vi "PIDF.vi"(4 "reinitialize? (F)":bool, 5 "invert? (F)":bool, 6 "PIDF gains":cluster{"Kp":dbl, "Ki":dbl, "Kd":dbl, "Kf":dbl} {"Kf" format="%.3f"; "Kd" format="%.3f"; "Ki" format="%.3f"; "Kp" format="%.3f"}, 7 "output range":cluster{"output high":dbl, "output low":dbl}={"output high"=1.0, "output low"=-1.0} {"output low" format="%.2f"; "output high" format="%.2f"}, 8 "i Zone":dbl=inf format="%.2f", 10 "process variable":dbl format="%.2f", 11 "setpoint":dbl format="%.2f") -> (1 "In i Zone?":bool, 2 "In Range?":bool, 3 "output":dbl format="%.2f")   [LabVIEW 2016]
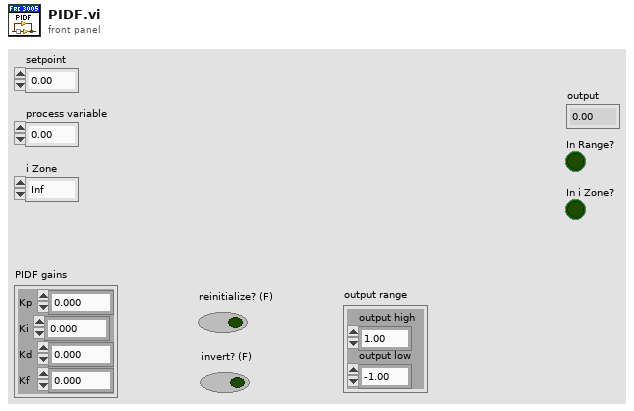
[diagram p1: front panel]
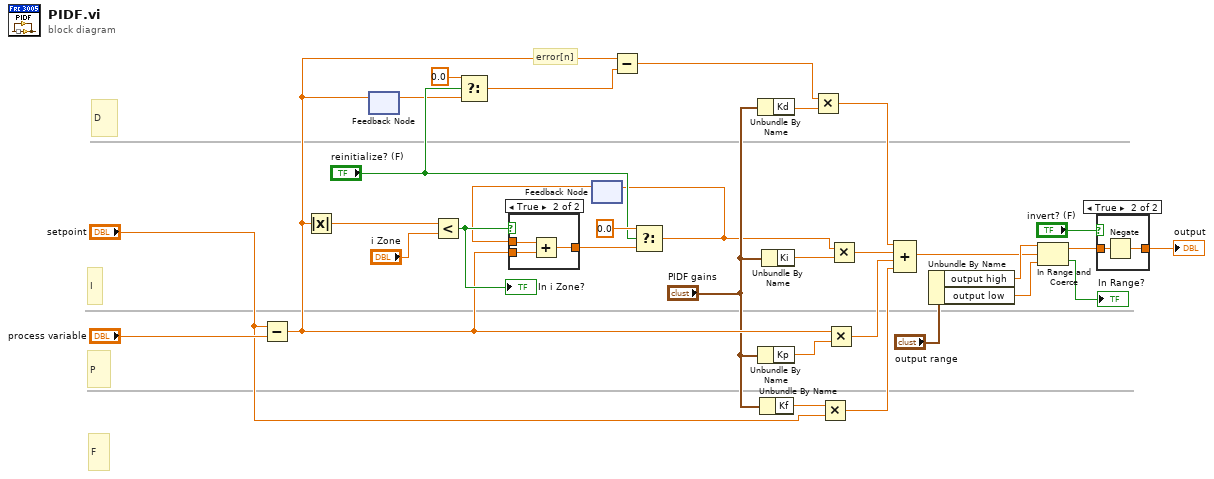
[diagram p0: block diagram]
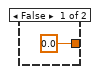
[diagram p3: hidden frame]
diagram:
  # "F"
  # "D"
  # "I"
  # "P"
  # "error[n]"
  n1 = Subtract(x="setpoint", y="process variable") -> (x-y=w23:dbl)
  n2 = Absolute Value(x=w23) -> (abs(x)=w30:dbl)
  n3 = feedback #1() -> (w21:dbl)  [unwired: 1 in]
  n4 = feedback-in #1(w23) -> ()
  n5 = Less?(x=w30, y="i Zone") -> (x < y?=w28:bool)
  "In i Zone?" <- w28
  n6 = Select(t=0.0 ("f"), s="reinitialize? (F)", f=w21) -> (s? t:f=w20:dbl)
  n7 = feedback #2() -> (w27:dbl)  [unwired: 1 in]
  n8 = case shown="True" w28 {
    tunnel: w23 -> [_ w36]
    tunnel: [0.0 ("f") w35] -> w26
    tunnel: w27 -> [_ w34]
    frame False {
    }
    frame True {
      n9 = Add(x=w34, y=w36) -> (x+y=w35:dbl)
    }
  }
  n10 = Subtract(x=w23, y=w20) -> (x-y=w10:dbl)
  n11 = Select(t=0.0 ("f"), s="reinitialize? (F)", f=w26) -> (s? t:f=w7:dbl)
  n12 = feedback-in #2(w7) -> ()
  n13 = Unbundle By Name("PIDF gains") -> ("Kd"=w11:dbl)
  n14 = Unbundle By Name("PIDF gains") -> ("Kp"=w31:dbl)
  n15 = Unbundle By Name("PIDF gains") -> ("Kf"=w13:dbl)
  n16 = Unbundle By Name("PIDF gains") -> ("Ki"=w8:dbl)
  n17 = Multiply(x=w10, y=w11) -> (x*y=w9:dbl)
  n18 = Multiply(x=w13, y="setpoint") -> (x*y=w12:dbl)
  n19 = Multiply(x=w23, y=w31) -> (x*y=w19:dbl)
  n20 = Multiply(x=w7, y=w8) -> (x*y=w6:dbl)
  n21 = Compound Arithmetic op=ADD(w9, w6, w19, w12) -> (w15:dbl)
  n22 = Unbundle By Name("output range") -> ("output high"=w17:dbl, "output low"=w16:dbl)
  n23 = In Range and Coerce(upper limit=w17, x=w15, lower limit=w16) -> (coerced(x)=w4:dbl, In Range?=→"In Range?":bool)
  n24 = case shown="True" "invert? (F)" {
    tunnel: w4 -> [w37 w39]
    tunnel: [w37 w38] -> w3
    frame False {
    }
    frame True {
      n25 = Negate(x=w39) -> (-x=w38:dbl)
    }
  }
  "output" <- w3
